vi "Obtain Tree Manager.vi"(8 "Error In":errorcluster) -> (0 "Error Out":errorcluster, 3 "Tree Manager":T1)   [LabVIEW 2016, in "Tree Manager.lvclass"]
doc: "Obtain a reference to the Tree Manager. If this is the first reference initialize the Manager."
uses:
  Tree Manager.lvclass
  Typedefs/Session Handle.ctl
  Data Types/Bool/Bool.lvclass
  C:/Users/plkruczp/Google Drive/MyCode/Modules/Tree/Tree Data/Tree Data.lvclass
  Data Types/Float/Float.lvclass
  Data Types/Int/Integer.lvclass
  Data Types/Path/Path.lvclass
  Data Types/String/String.lvclass
  Tree Manager.lvclass/Tree Manager.ctl
  Tree Data/Tree Data.lvclass
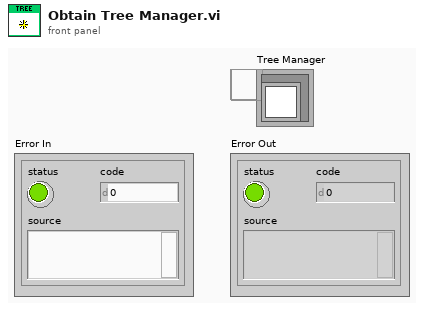
[diagram p1: front panel]
types:
  T1 = typedef "Tree Manager.lvclass/Session Handle.ctl" = refnum<data-value>
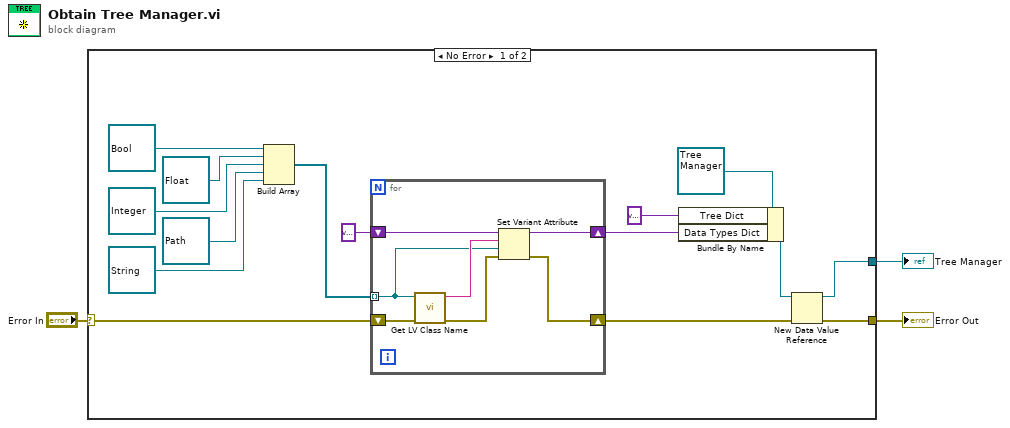
[diagram p0: block diagram]
diagram:
  n1 = case shown="No Error" "Error In" {
    selector: "Error In" -> [w8 w26]
    tunnel: [w4 w26] -> w1
    tunnel: [w5 _] -> w3
    frame No Error {
      n2 = Build Array(refnum<class "Bool.lvclass"> refnum ("Bool.lvclass"), refnum<class "Float.lvclass"> refnum ("Float.lvclass"), refnum<class "Integer.lvclass"> refnum ("Int.lvclass"), refnum<class "Path.lvclass"> refnum ("Path.lvclass"), refnum<class "String.lvclass"> refnum ("String.lvclass")) -> (w9:refnum<class "Tree Data.lvclass">[])
      n3 = for {
        shift-right: [w24] -> w11
        shift-left: variant ("Tree Dictionary") -> [w25]
        tunnel: w9 -> [w22] mode=indexing
        shift-right: [w19] -> w7
        shift-left: w8 -> [w21]
        n4 = call <vilib>:"Get LV Class Name.vi"("error in (no error)"=w21, "object"=w22) -> ("error out"=w20:errorcluster, "class name"=w23:string)  [unwired: 8 in]
        n5 = Set Variant Attribute(Variant=w25, name=w23, value=w22, error in=w20) -> (Variant out=w24:variant, error out=w19:errorcluster)  [unwired: 1 out]
      }
      n6 = Bundle By Name(cluster=refnum<class "Tree Manager.lvclass"> refnum, "Tree Dict"=variant ("Tree Dictionary"), "Data Types Dict"=w11) -> (w6:refnum<class "Tree Manager.lvclass">)
      n7 = New Data Value Reference(data value=w6, error in=w7) -> (data value reference=w5:refnum<data-value>, error out=w4:errorcluster)
    }
    frame Error {
    }
  }
  "Tree Manager" <- w3
  "Error Out" <- w1
